vi "DrawRectExample.vi"() -> ()   [LabVIEW 2010]
panel:
  out "picture":picture
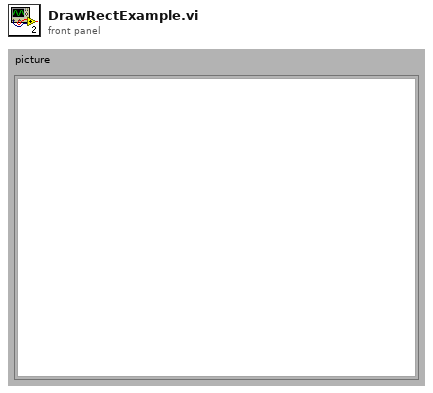
[diagram p1: front panel]
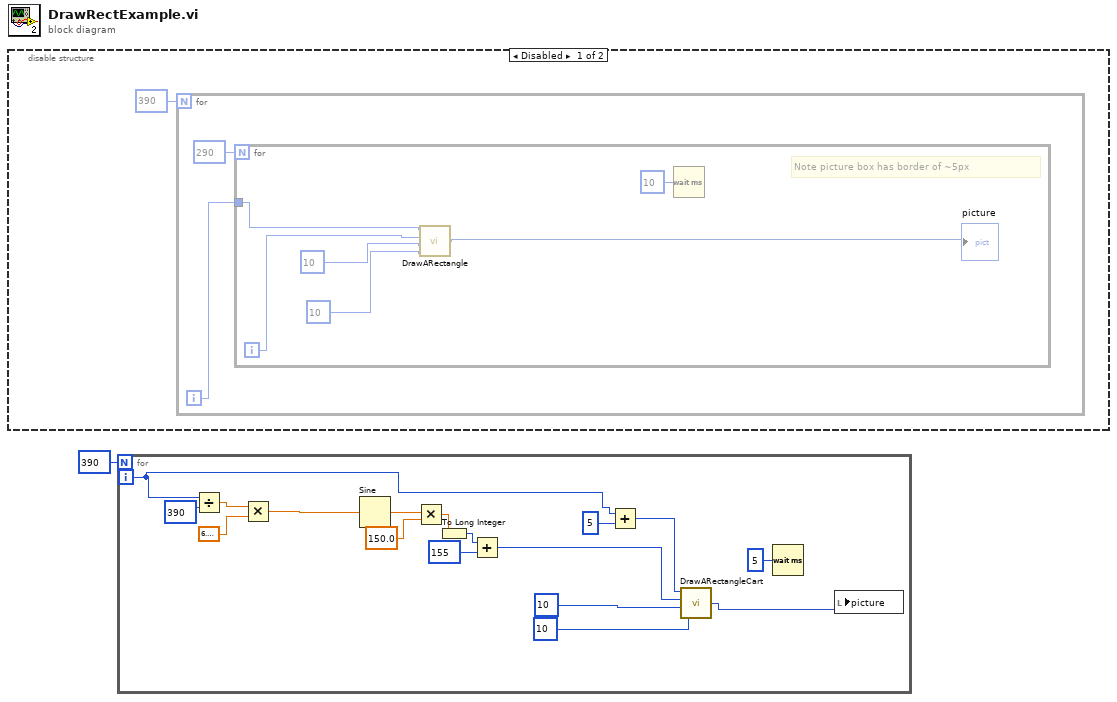
[diagram p0: block diagram]
diagram:
  n1 = disable-structure shown="Disabled" {
    frame Disabled {
      n2 = for {
        N: 390 -> [_]
        i -> [w3]
        n3 = for {
          N: 290 -> [_]
          tunnel: w3 -> [w10]
          i -> [w9]
          # "Note picture box has border of ~5px"
          n4 = call "DrawARectangle.vi"("height"=10, "width"=10, "y"=w9, "x"=w10) -> ("picture"=→"picture":picture)
          n5 = Wait (ms)(milliseconds to wait=u32 10) -> ()  [unwired: 1 out]
        }
      }
    }
    frame Enabled {
    }
  }
  n6 = for {
    N: 390 -> [_]
    i -> [w13]
    n7 = Divide(x=w13, y=390) -> (x/y=w16:dbl)
    n8 = Multiply(x=w16, y=6.283185307179586) -> (x*y=w15:dbl)
    n9 = Sine(x=w15) -> (sin(x)=w25:dbl)
    n10 = Multiply(x=w25, y=150.0) -> (x*y=w23:dbl)
    n11 = To Long Integer(number=w23) -> (32bit integer=w22:i32)
    n12 = Add(x=w22, y=155) -> (x+y=w26:i32)
    n13 = Add(x=w13, y=5) -> (x+y=w12:i32)
    n14 = call "DrawARectangleCart.vi"("height"=10, "width"=10, "y"=w26, "x"=w12) -> ("picture"=w18:picture)
    n15 = Wait (ms)(milliseconds to wait=u32 5) -> ()  [unwired: 1 out]
    n16 = local write "picture"(w18) -> ()
  }
